vi "filterVMax.vi"(0 "Game in":refnum<class "Game.lvclass">, 1 "safeDriveVel":dbl=0.4 format="%#_13g", 3 "KepperMaxVSent":dbl, 4 "MaxVSent":dbl, 5 "error in (no error)":errorcluster, 6 "StopVelocity":dbl, 7 "MaxVAng":dbl, 8 "MaxStopVAng":dbl, 10 "VelocityInDirects":dbl, 11 "Robot in":refnum<class "Robot.lvclass">) -> (14 "Game out":refnum<class "Game.lvclass">, 15 "MaxVSent out":dbl, 18 "MaxVAng out":dbl, 19 "error out":errorcluster)   [LabVIEW 2021, in "Game.lvclass"]
uses:
  Game.lvclass
  Robot_class/Robot.lvclass
  D:/RoboIme/horie/SSL_AI/Object_class/Object.lvclass
  Referee_class/command_interpreted.ctl
  Navigation/driveMode.ctl
  Game.lvclass/Game.ctl
  Parameters_class/Parameters.lvclass/Parameters.ctl
  Team_class/Team.lvclass/Team.ctl
  Referee_class/Referee.lvclass/Referee.ctl
  Events_class/Events.lvclass/Events.ctl
  Robot_class/Robot.lvclass/Robot.ctl
  Object_class/Object.lvclass/Object.ctl
  Parameters_class/Read DistanceStop.vi
  Read BallRef.vi
  Object_class/Read position(x,y).vi
  Robot_class/Read robotKickState.vi
  Robot_class/Read tactic.vi
  Robot_class/Read id.vi
  Read Referee.vi
  Read EventsRef.vi
  Events_class/Read ball_out.vi
  Referee_class/Read command_interpreted.vi
  Referee_class/Read our_goalie_id.vi
  Read Parameters.lvclass.vi
  Read NewParameters.vi
  Read EnemyRef.vi
  Team_class/Read RobotRef.vi
  Parameters_class/Read bangBangParameters.vi
  Enemy_class/Enemy.lvclass
  D:/RoboIme/horie/SSL_AI/Team_class/Team.lvclass
  Ball_class/Ball.lvclass
  Parameters_class/Parameters.lvclass
  Referee_class/Referee.lvclass
  Events_class/Events.lvclass
  Utilities_class/Utilities.lvclass
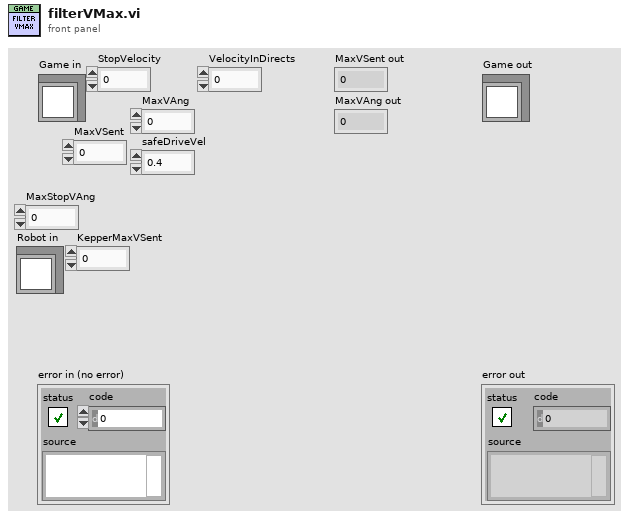
[diagram p1: front panel]
types:
  T1 = typedef "command_interpreted.ctl" = enum16{"Goal Ally", "Goal Enemy", "Ball Placement Enemy", "Ball Placement Ally", "Normal Half Time", "Extra Time  Break", "Extra Half Time", "None", "Post Game", "PKA Normal Start", "Prepare Kickoff Ally", "PKE Normal Start", "Prepare Kickoff Enemy", "Force Start", "Halt", "Timeout", "Prepare Penalty Ally", "Prepare Penalty Enemy", "PPA NormalStart", "PPE Normal Start", "Indirect Free Ally", "Direct Free Enemy", "Direct Free Ally", "Indirect Free Enemy", "Stop"}
  T2 = typedef "driveMode.ctl" = enum16{"Fast", "SafeDrive"}
  T3 = typedef "NewParameters.ctl" = cluster{"PenaltyDistance":dbl, "DistanceAttackerToBackBall":dbl, "Division":enum16{"Div B", "Div A"}, "DistanceToAvoidyEnemyRobot":dbl, "BallPlacementDistance":dbl, "DisatanceBehindBallToStealBall":dbl, "MaxDistanceToPositionKickoff":dbl, "BlockEnemyTarget":bool, "MaxStopVAng":dbl, "DistanceMarkerToEnemy":dbl, "IgnoreDribblerContact":bool, "DistanceToBeginEnemyPosession":dbl, "GoToBallWhenEnemyNotMoving":bool, "EnemyDistanceToReduceVelocity":dbl, "TurnOnEnemyDistanceToReduceVelocity":bool, "EnemyDistanceToShootOutBall":dbl, "DefenseKickBall":bool, "MoreKickToGoal? (0-0.3)":dbl, "ChipKickInEnemyField":bool, "ShootOutRobotId":dbl, "FieldLenghtDenominatorInShootOut":dbl, "AdjustPositionInBallPlacement":bool, "PowerGodPass":dbl, "VelocityAbortEnemyPos":dbl, "MaxDistToBeginPass":dbl, "MinDistToBeginPass":dbl, "VelocityInDirects":dbl, "BadDribblerIDs":i32[], "NewKickToDistanceAroundBall":dbl, "PowerAvoidColisionMarker":dbl, "DistanceToAvoidColisionMarker":dbl, "AvoidBallKick":dbl, "DistanceTryKick":dbl, "SuicideKickDIstance":dbl, "FirstKickAtck":bool, "AdjustFirstKickDistance":dbl, "FirstKickDefense":bool, "AvoidAimLessKick":dbl, "DistanceToAvoidyEnemyShootRobot ":dbl, "NumberOfMarkers":dbl, "PotField":bool, "PIDLateral":bool, "MinDistanceFirstKickX":dbl, "MinDistanceFirstKickY":dbl, "FractionOfDistToTouchGround\nAfterChipKick":dbl, "FractionOfKickxWhen\nComposedWithKickz":dbl, "Style":T4, "MoveInTurnState":bool, "DistFromEnemyToConsider\nMoveInTurnState":dbl, "CascadePID":bool, "TurnAroundParameters":cluster{"Radius":dbl, "Multiplier":dbl, "ChordAngle":dbl}, "SafeDriveVel":dbl}
  T4 = typedef "Style.ctl" = enum16{"Insanity", "Offensive", "Defensive"}
  T5 = typedef "tactics.ctl" = enum16{"GoToBallPlacementPosition", "PlaceBall", "GoToBallPlacement", "5Robots", "BallPlacementEnemy", "ReceivePassInFuturePoint", "Roller", "PrepareRollToPassRollerGoTo", "PrepareRollToPassReceiverGoTo", "WaitRoll", "PositionToRoll", "PenaltyAttacker", "PassObserver", "PenaltyDefense", "TableReceiverTactic", "Test", "DefendGoal", "Marker", "FollowAttacker", "DefendArea", "Shoot", "AttackerAimGoal", "AttackerBallOutOfField", "AttackerBlock", "AttackerStop", "Duelist", "Halt", "ZigZag", "GoTo", "Timeout", "KickToBestRobot", "KickToPassReceiver", "PositionToReceivePass", "WaitPass"}
  T6 = typedef "robotKickToStates.ctl" = enum16{"shootFromDirect", "avoidCollideBall", "goToBackBall", "none", "walk", "turn", "oldKickToShoot", "oldKickToGoToBackBall", "shoot"}
  T7 = typedef "bangBangControlParameters.ctl" = cluster{"MaxVSent":dbl, "MaxVNorm":dbl, "MaxVAng":dbl, "VAngCircle":dbl, "LBeginCircle":dbl, "DistToDestOrientation":dbl, "MaxVAngToTurn":dbl, "AtkDistToDestOrientation":dbl, "KepperMaxVSent":dbl, "VelNearEnemy":dbl}
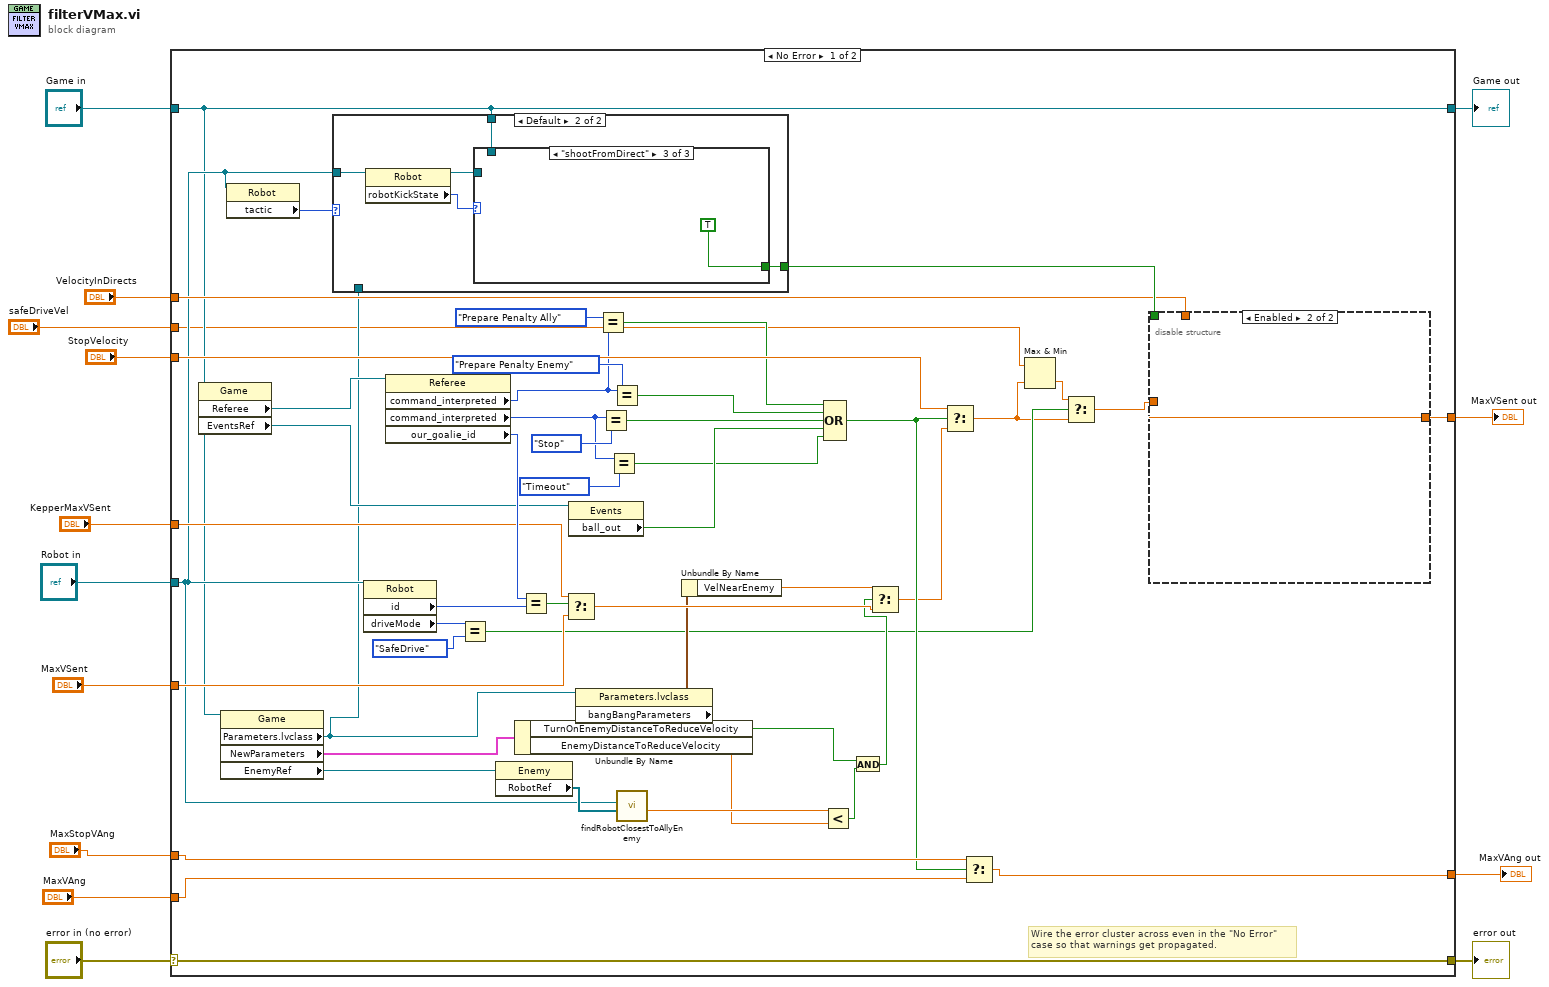
[diagram p0: block diagram]
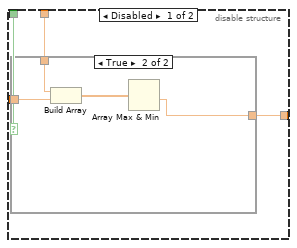
[diagram p2: hidden frame]
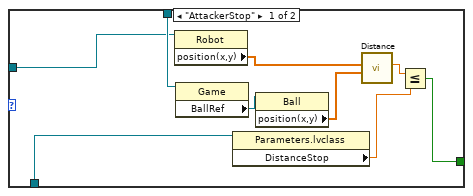
[diagram p4: hidden frame]
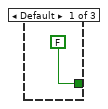
[diagram p5: hidden frame]
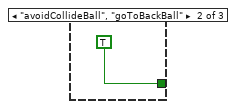
[diagram p6: hidden frame]
diagram:
  n1 = case shown="No Error" "error in (no error)" {
    selector: "error in (no error)" -> [w64 w93]
    tunnel: [w64 w93] -> w13
    tunnel: [w26 w92] -> w11
    tunnel: "Game in" -> [w26 w92]
    tunnel: "MaxVSent" -> [w50 _]
    tunnel: "StopVelocity" -> [w62 _]
    tunnel: "MaxStopVAng" -> [w61 _]
    tunnel: "MaxVAng" -> [w60 _]
    tunnel: [w59 _] -> w6
    tunnel: "Robot in" -> [w28 _]
    tunnel: "KepperMaxVSent" -> [w49 _]
    tunnel: [w32 _] -> w3
    tunnel: "VelocityInDirects" -> [w31 _]
    tunnel: "safeDriveVel" -> [w20 _]
    frame No Error {
      # "Wire the error cluster across even in the \"No Error\"\ncase so that warnings get propagated."
      n2 = property class="Game"(reference=w26) -> ("Referee"=w30:refnum<class "Referee.lvclass">, "EventsRef"=w29:refnum<class "Events.lvclass">)  [unwired: 1 in, 2 out]
      n3 = property class="Game"(reference=w26) -> ("Parameters.lvclass"=w25:refnum<class "Parameters.lvclass">, "NewParameters"=w45:T3, "EnemyRef"=w48:refnum<class "Enemy.lvclass">)  [unwired: 1 in, 2 out]
      n4 = property class="Robot"(reference=w28) -> ("tactic"=w27:T5)  [unwired: 1 in, 2 out]
      n5 = case shown="Default" w27 {
        tunnel: w28 -> [w77 w88]
        tunnel: [w83 w86] -> w33
        tunnel: w26 -> [w82 w84]
        tunnel: w25 -> [w76 _]
        frame "AttackerStop" {
          n6 = property class="Robot"(reference=w77) -> ("position(x,y)"=w81:dbl[])  [unwired: 1 in, 2 out]
          n7 = property class="Game"(reference=w82) -> ("BallRef"=w80:refnum<class "Ball.lvclass">)  [unwired: 1 in, 2 out]
          n8 = property class="Parameters.lvclass"(reference=w76) -> ("DistanceStop"=w75:dbl)  [unwired: 1 in, 2 out]
          n9 = property class="Ball"(reference=w80) -> ("position(x,y)"=w79:dbl[])  [unwired: 1 in, 2 out]
          n10 = call "Distance.vi"("P1"=w79, "P2"=w81) -> ("Distance"=w78:dbl)  [unwired: 7 in, 2 out]
          n11 = Less Or Equal?(x=w78, y=w75) -> (x <= y?=w83:bool)
        }
        frame Default {
          n12 = property class="Robot"(reference=w88) -> (reference out=w85:refnum<class "Robot.lvclass">, "robotKickState"=w87:T6)  [unwired: 1 in, 1 out]
          n13 = case shown="\"shootFromDirect\"" w87 {
            tunnel: [FALSE TRUE TRUE] -> w86
            tunnel: w85 -> [_ _ _]
            tunnel: w84 -> [_ _ _]
            frame Default {
            }
            frame "avoidCollideBall", "goToBackBall" {
            }
            frame "shootFromDirect" {
            }
          }
        }
      }
      n14 = property class="Robot"(reference=w28) -> ("id"=w53:i32, "driveMode"=w24:T2)  [unwired: 1 in, 2 out]
      n15 = property class="Referee"(reference=w30) -> ("command_interpreted"=w36:T1, "command_interpreted"=w16:T1, "our_goalie_id"=w52:i32)  [unwired: 1 in, 2 out]
      n16 = Equal?(x=w24, y=driveMode."SafeDrive") -> (x = y?=w22:bool)
      n17 = property class="Enemy"(reference=w48) -> ("RobotRef"=w47:refnum<class "Robot.lvclass">[])  [unwired: 1 in, 2 out]
      n18 = Unbundle By Name(w45) -> ("TurnOnEnemyDistanceToReduceVelocity"=w40:bool, "EnemyDistanceToReduceVelocity"=w44:dbl)
      n19 = Equal?(x=w52, y=w53) -> (x = y?=w51:bool)
      n20 = Select(t=w49, s=w51, f=w50) -> (s? t:f=w43:dbl)
      n21 = property class="Events"(reference=w29) -> ("ball_out"=w57:bool)  [unwired: 1 in, 2 out]
      n22 = property class="Parameters.lvclass"(reference=w25) -> ("bangBangParameters"=w38:T7)  [unwired: 1 in, 2 out]
      n23 = Equal?(x=command_interpreted."Prepare Penalty Ally", y=w36) -> (x = y?=w34:bool)
      n24 = Equal?(x=w16, y=command_interpreted."Stop") -> (x = y?=w56:bool)
      n25 = Equal?(x=w16, y=command_interpreted."Timeout") -> (x = y?=w15:bool)
      n26 = Equal?(x=w36, y=command_interpreted."Prepare Penalty Enemy") -> (x = y?=w54:bool)
      n27 = call "findRobotClosestToAllyEnemy.vi"("Ally/Enemy Robots"=w47, "Robot Target"=w28) -> ("Robot distance to other one"=w46:dbl)  [unwired: 6 in, 3 out]
      n28 = Unbundle By Name(w38) -> ("VelNearEnemy"=w37:dbl)
      n29 = Less?(x=w46, y=w44) -> (x < y?=w41:bool)
      n30 = Compound Arithmetic op=OR(w34, w54, w56, w57, w15) -> (w58:bool)
      n31 = And(x=w40, y=w41) -> (x .and. y?=w39:bool)
      n32 = Select(t=w37, s=w39, f=w43) -> (s? t:f=w42:dbl)
      n33 = Select(t=w62, s=w58, f=w42) -> (s? t:f=w19:dbl)
      n34 = Select(t=w61, s=w58, f=w60) -> (s? t:f=w59:dbl)
      n35 = Max & Min(x=w20, y=w19) -> (min(x,y)=w18:dbl)  [unwired: 1 out]
      n36 = Select(t=w18, s=w22, f=w19) -> (s? t:f=w21:dbl)
      n37 = disable-structure shown="Enabled" {
        disable-tunnel: w33 -> [w68 _]
        disable-tunnel: w21 -> [w67 w74]
        disable-tunnel: [w66 w74] -> w32
        disable-tunnel: w31 -> [w65 _]
        frame Disabled {
          n38 = case shown="True" w68 {
            tunnel: w67 -> [w69 w73]
            tunnel: [w69 w71] -> w66
            tunnel: w65 -> [_ w70]
            frame False {
            }
            frame True {
              n39 = Build Array(w70, w73) -> (w72:dbl[])
              n40 = Array Max & Min(array=w72) -> (min value=w71:dbl)  [unwired: 3 out]
            }
          }
        }
        frame Enabled {
        }
      }
    }
    frame Error {
    }
  }
  "error out" <- w13
  "Game out" <- w11
  "MaxVSent out" <- w3
  "MaxVAng out" <- w6
